vi "prepare_inserts_for_save_audit_results.vi"(7 "audit_id":i32, 8 "error_in":errorcluster, 10 "results_from_PLC":T1, 11 "archivisation_info":string[][](array[string])) -> (0 "error_out":errorcluster, 3 "INSERT_statements":string[](array[string]))   [LabVIEW 2020]
uses:
  ST_results_info.ctl
  _misc/AULocalize/SubVIs/Get Localized Phrase Compact Interface 0D.vi
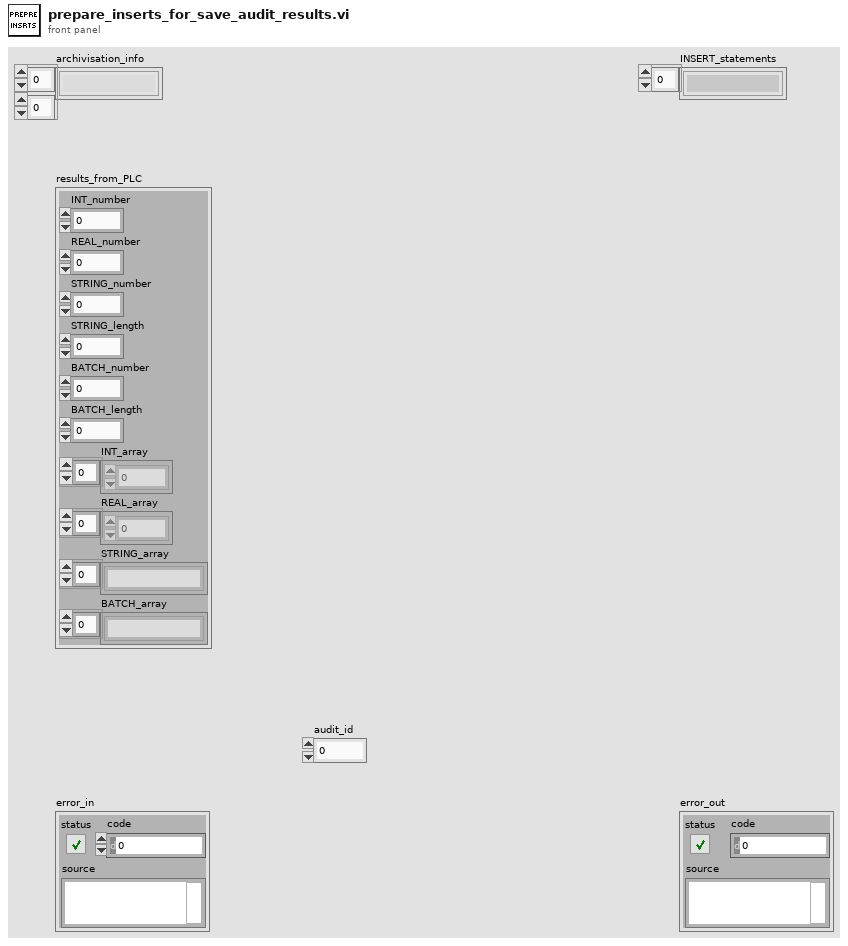
[diagram p1: front panel]
types:
  T1 = typedef "ST_results_info.ctl" = cluster{"INT_number":i32, "REAL_number":i32, "STRING_number":i32, "STRING_length":i32, "BATCH_number":i32, "BATCH_length":i32, "INT_array":i16[], "REAL_array":sgl[], "STRING_array":string[], "BATCH_array":string[]}
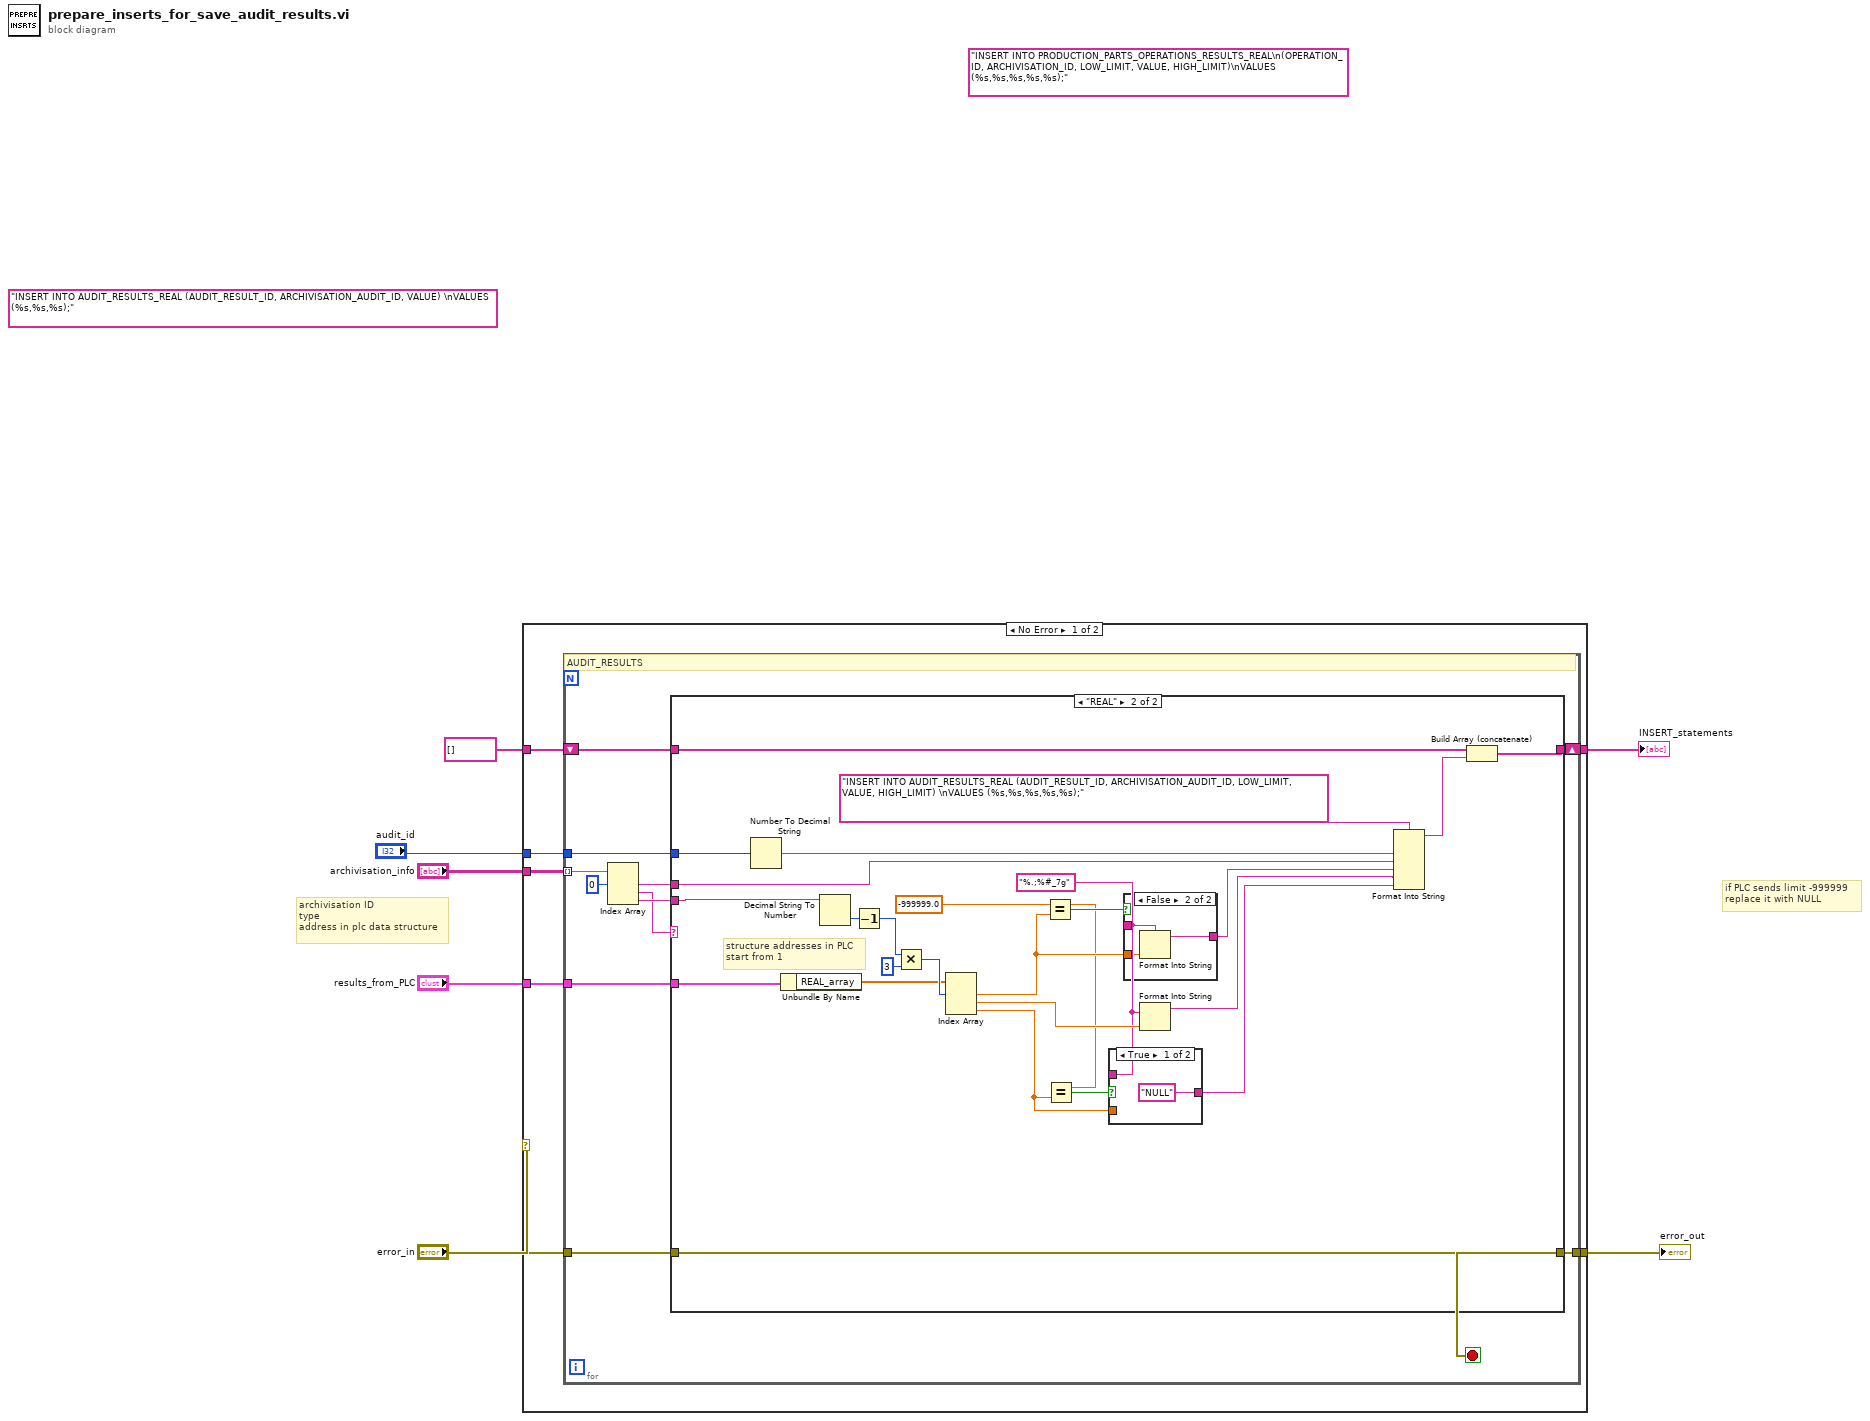
[diagram p0: block diagram]
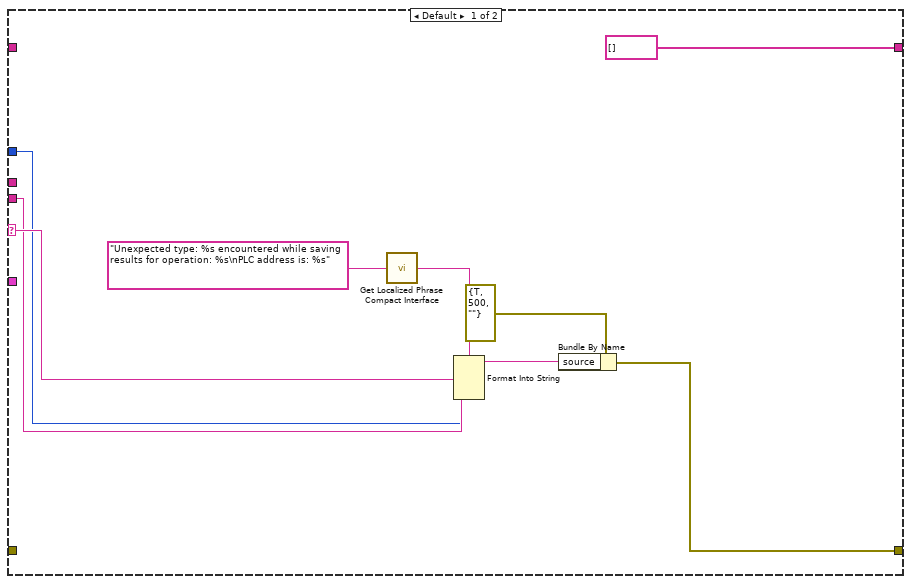
[diagram p2: hidden frame]
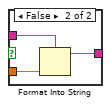
[diagram p3: hidden frame]
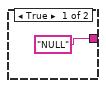
[diagram p4: hidden frame]
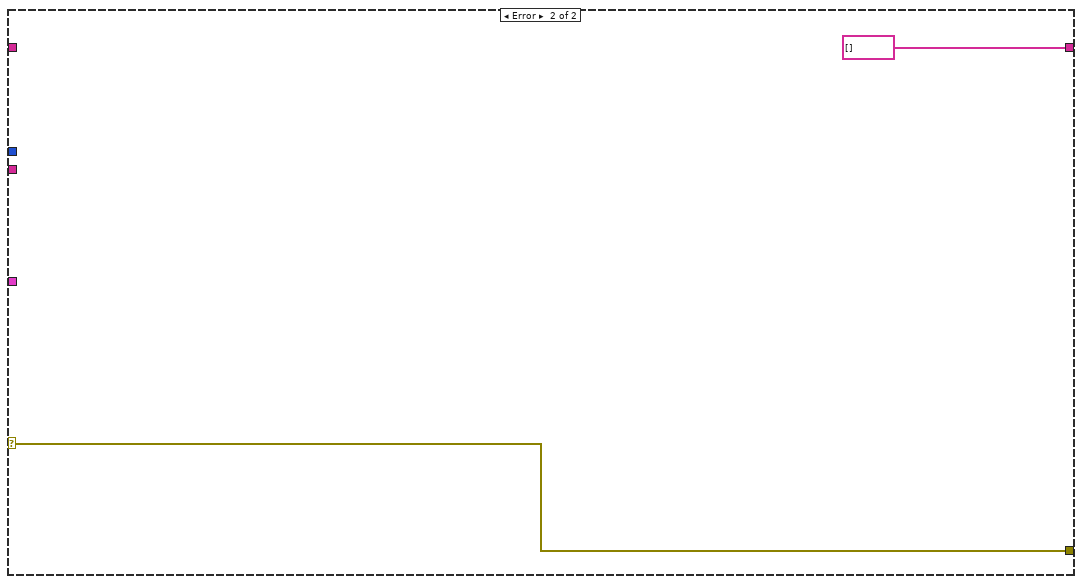
[diagram p5: hidden frame]
diagram:
  (unwired) "INSERT INTO AUDIT_RESULTS_REAL (AUDIT_RESULT_ID, ARCHIVISATION_AUDIT_ID, VALUE) \nVALUES (%s,%s,%s);"
  (unwired) "INSERT INTO PRODUCTION_PARTS_OPERATIONS_RESULTS_REAL\n(OPERATION_ID, ARCHIVISATION_ID, LOW_LIMIT, VALUE, HIGH_LIMIT)\nVALUES (%s,%s,%s,%s,%s);"
  # "if PLC sends limit -999999\nreplace it with NULL"
  # "archivisation ID\ntype\naddress in plc data structure"
  n1 = case shown="No Error" "error_in" {
    selector: "error_in" -> [w12 w69]
    tunnel: "archivisation_info" -> [w14 _]
    tunnel: string[] [] ("INSERT_statements") -> [w13 _]
    tunnel: [w10 string[] [] ("INSERT_statements")] -> w5
    tunnel: "results_from_PLC" -> [w11 _]
    tunnel: "audit_id" -> [w8 _]
    tunnel: [w9 w69] -> w2
    frame No Error {
      n2 = for {
        tunnel: w14 -> [w23] mode=indexing
        shift-right: [w24] -> w10
        shift-left: w13 -> [w25]
        tunnel: w11 -> [w19]
        tunnel: w8 -> [w20]
        tunnel: w12 -> [w16]
        tunnel: [w15] -> w9
        stop <- w15 stop-if-true
        # "AUDIT_RESULTS"
        n3 = Index Array(array=w23, index #1=0 ("index")) -> (element #1=w21:string, element #2=w17:string, element #3=w18:string)  [unwired: 2 in]
        n4 = case shown="\"REAL\"" w17 {
          selector: w17 -> [w30 _]
          tunnel: w25 -> [_ w59]
          tunnel: [string[] [] w58] -> w24
          tunnel: w21 -> [_ w55]
          tunnel: w20 -> [w27 w53]
          tunnel: w19 -> [_ w38]
          tunnel: w18 -> [w28 w39]
          tunnel: w16 -> [_ w54]
          tunnel: [w32 w54] -> w15
          frame Default {
            n5 = call-poly "Get Localized Phrase Compact Interface.vi"("Key"="Unexpected type: %s encountered while saving results for operation: %s\nPLC address is: %s" ("source")) -> ("Translated Phrase"=w26:string)
            n6 = Format Into String(format string=w26, w30, w27, w28) -> (resulting string=w31:string)  [unwired: 2 in, 1 out]
            n7 = Bundle By Name(cluster=errorcluster {"status"=TRUE, "code"=500, "source"=""} ("error IO"), "source"=w31) -> (w32:errorcluster)
          }
          frame "REAL" {
            w42 = "%.;%#_7g" ("format string")
            w41 = sgl -999999.0 ("x")
            # "structure addresses in PLC\nstart from 1"
            n8 = Number To Decimal String(number=w53) -> (decimal integer string=w52:string)  [unwired: 1 in]
            n9 = Unbundle By Name(w38) -> ("REAL_array"=w43:sgl[])
            n10 = Decimal String To Number(string=w39) -> (number=w49:i32)  [unwired: 2 in, 1 out]
            n11 = Decrement(x=w49) -> (x-1=w50:i32)
            n12 = Multiply(x=w50, y=3) -> (x*y=w44:i32)
            n13 = Index Array(array=w43, index #1=w44) -> (element #1=w46:sgl, element #2=w51:sgl, element #3=w48:sgl)  [unwired: 2 in]
            n14 = Equal?(x=w41, y=w46) -> (x = y?=w45:bool)
            n15 = Equal?(x=w41, y=w48) -> (x = y?=w47:bool)
            n16 = case shown="True" w47 {
              tunnel: ["NULL" w63] -> w35
              tunnel: w48 -> [_ w62]
              tunnel: w42 -> [_ w61]
              frame True {
              }
              frame False {
                n17 = Format Into String(format string=w61, w62) -> (resulting string=w63:string)  [unwired: 2 in, 1 out]
              }
            }
            n18 = case shown="False" w45 {
              tunnel: ["NULL" w66] -> w37
              tunnel: w46 -> [_ w67]
              tunnel: w42 -> [_ w65]
              frame True {
              }
              frame False {
                n19 = Format Into String(format string=w65, w67) -> (resulting string=w66:string)  [unwired: 2 in, 1 out]
              }
            }
            n20 = Format Into String(format string=w42, w51) -> (resulting string=w36:string)  [unwired: 2 in, 1 out]
            n21 = Format Into String(format string="INSERT INTO AUDIT_RESULTS_REAL (AUDIT_RESULT_ID, ARCHIVISATION_AUDIT_ID, LOW_LIMIT, VALUE, HIGH_LIMIT) \nVALUES (%s,%s,%s,%s,%s);", w52, w55, w37, w36, w35) -> (resulting string=w56:string)  [unwired: 2 in, 1 out]
            n22 = Build Array (concatenate)(w59, w56) -> (w58:string[])
          }
        }
      }
    }
    frame Error {
    }
  }
  "INSERT_statements" <- w5
  "error_out" <- w2
